vi "Compile Engine Data.vi"(8 "error in (no error)":errorcluster, 11 "Device Item Ref in":T1 format="%.0x") -> (0 "error out":errorcluster)   [LabVIEW 2023, in "NI 272x Resistive Simulation Custom Device Configuration.lvlib"]
uses:
  NI 272x Resistive Simulation Custom Device Configuration.lvlib
  <vilib>/NI VeriStand/Custom Device API/Custom Device Item Ref.ctl
  Controls/Compiled Engine Data.ctl
  Controls/Compiled HW Channel.ctl
  Controls/Channel Mode.ctl
  <instrlib>/ni272xReferenceVIs/ni272xReferenceVIs.llb/ni272x Callendar-Van Dusen RTD Parameters.ctl
  Controls/Compiled Connect Channel.ctl
  Globals/Names.vi
  <vilib>/NI VeriStand/Custom Device Tools/Custom Device Utility Library/NI VeriStand - Search for Item by Name.vi
  <vilib>/NI VeriStand/Custom Device API/Get Item Property (String).vi
  <vilib>/NI VeriStand/Custom Device API/Get Item Property (Double).vi
  <vilib>/NI VeriStand/Custom Device API/Set Item Property (Variant).vi
  <vilib>/NI VeriStand/Custom Device Tools/Custom Device Utility Library/Custom Device Utility Library.lvlib
  <vilib>/NI VeriStand/Custom Device API/Custom Device API.lvlib
  NI 272x Resistive Simulation Custom Device Shared.lvlib
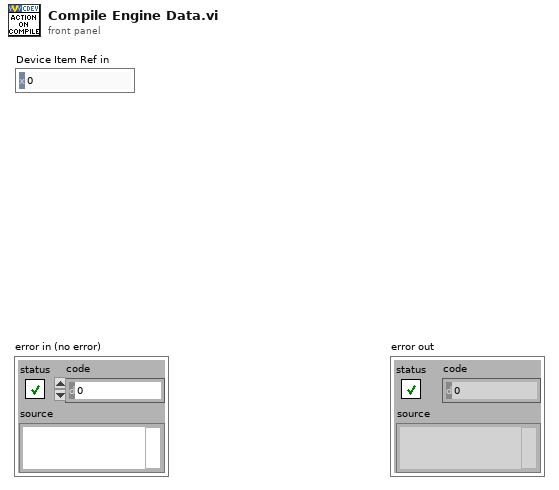
[diagram p1: front panel]
types:
  T1 = typedef "Custom Device API.lvlib/Custom Device Item Ref.ctl" = u64
  T2 = typedef "NI 272x Resistive Simulation Custom Device Shared.lvlib/Compiled Engine Data.ctl" = cluster{"HW Chns":T3[], "Con Chns":T6[], "Err Idx":i32, "Late Idx":i32, "Dur Idx":i32, "DevName":string, "CD In Size":i32, "CD Out Size":i32, "TL dt":i64}
  T3 = typedef "NI 272x Resistive Simulation Custom Device Shared.lvlib/Compiled HW Channel.ctl" = cluster{"Mode":T4, "RTD":T5, "Desired Idx":i32, "Actual Idx":i32, "Last Des Val":dbl, "HW CH":string}
  T4 = typedef "NI 272x Resistive Simulation Custom Device Shared.lvlib/Channel Mode.ctl" = enum16{"Resistance", "RTD Temperature"}
  T5 = typedef "ni272x Callendar-Van Dusen RTD Parameters.ctl" = cluster{"A":dbl, "B":dbl, "C":dbl, "R0":dbl}
  T6 = typedef "NI 272x Resistive Simulation Custom Device Shared.lvlib/Compiled Connect Channel.ctl" = cluster{"Chn Idx":i32, "HW CH":string, "Is Con":bool, "HW CH+1":string}
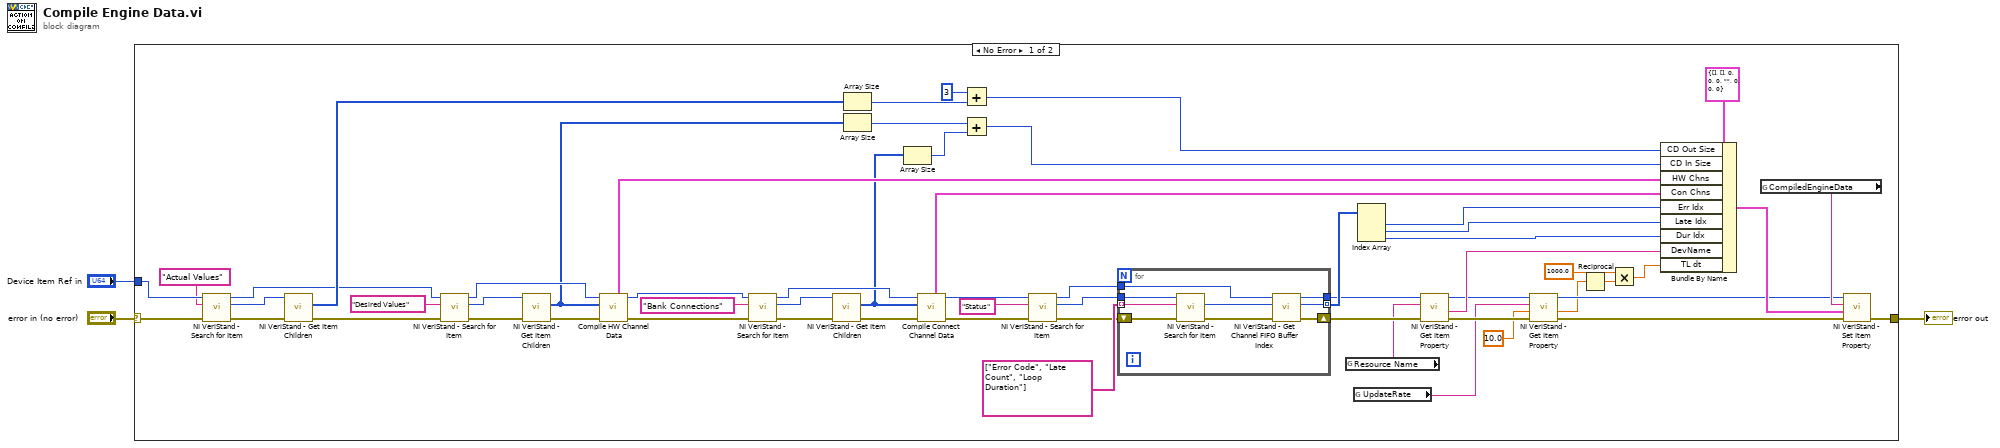
[diagram p0: block diagram]
diagram:
  n1 = case shown="No Error" "error in (no error)" {
    selector: "error in (no error)" -> [w62 w72]
    tunnel: [w34 w72] -> w2
    tunnel: "Device Item Ref in" -> [w10 _]
    frame No Error {
      n2 = call-poly <vilib>:"NI VeriStand - Search for Item.vi"("error in"=w62, "Item Name"="Actual Values", "Section Ref in"=w10) -> ("error out"=w11:errorcluster, "Item Ref"=w5:T1, "Section Ref out"=w4:T1)  [unwired: 5 in, 1 out]
      n3 = call <vilib>:"NI VeriStand - Get Item Children.vi"("error in (no error)"=w11, "Item Ref in"=w5) -> ("error out"=w8:errorcluster, "Child Refs"=w7:T1[])  [unwired: 6 in, 2 out]
      n4 = call-poly <vilib>:"NI VeriStand - Search for Item.vi"("error in"=w8, "Item Name"="Desired Values", "Section Ref in"=w4) -> ("error out"=w60:errorcluster, "Item Ref"=w59:T1, "Section Ref out"=w57:T1)  [unwired: 5 in, 1 out]
      n5 = call <vilib>:"NI VeriStand - Get Item Children.vi"("error in (no error)"=w60, "Item Ref in"=w59) -> ("error out"=w58:errorcluster, "Child Refs"=w27:T1[])  [unwired: 6 in, 2 out]
      n6 = call "Compile HW Channel Data.vi"("error in (no error)"=w58, "Desired Values Refs"=w27, "Device ref"=w57) -> ("error out"=w53:errorcluster, "Device ref dup"=w52:T1, "Compiled HW Channels"=w55:T3[])  [unwired: 6 in]
      n7 = call-poly <vilib>:"NI VeriStand - Search for Item.vi"("error in"=w53, "Item Name"="Bank Connections", "Section Ref in"=w52) -> ("error out"=w51:errorcluster, "Item Ref"=w49:T1, "Section Ref out"=w48:T1)  [unwired: 5 in, 1 out]
      n8 = call <vilib>:"NI VeriStand - Get Item Children.vi"("error in (no error)"=w51, "Item Ref in"=w49) -> ("error out"=w50:errorcluster, "Child Refs"=w26:T1[])  [unwired: 6 in, 2 out]
      n9 = Array Size(array=w7) -> (size(s)=w6:i32)
      n10 = Array Size(array=w27) -> (size(s)=w25:i32)
      n11 = Array Size(array=w26) -> (size(s)=w24:i32)
      n12 = call "Compile Connect Channel Data.vi"("error in (no error)"=w50, "Connect Chan Refs"=w26, "Device ref"=w48) -> ("error out"=w46:errorcluster, "Device ref dup"=w45:T1, "Compiled HW Channels"=w47:T6[])  [unwired: 6 in]
      n13 = Add(x=3, y=w6) -> (x+y=w21:i32)
      n14 = Add(x=w25, y=w24) -> (x+y=w23:i32)
      n15 = call-poly <vilib>:"NI VeriStand - Search for Item.vi"("error in"=w46, "Item Name"="Status", "Section Ref in"=w45) -> ("error out"=w42:errorcluster, "Item Ref"=w41:T1, "Section Ref out"=w40:T1)  [unwired: 5 in, 1 out]
      n16 = for {
        tunnel: string[] ["Error Code", "Late Count", "Loop Duration"] -> [w71] mode=indexing
        tunnel: w41 -> [w69]
        shift-right: [w65] -> w35
        shift-left: w42 -> [w70]
        tunnel: w40 -> [w67]
        tunnel: [w64] -> w39 mode=indexing
        tunnel: [w63] -> w30
        n17 = call-poly <vilib>:"NI VeriStand - Search for Item.vi"("error in"=w70, "Item Name"=w71, "Section Ref in"=w69) -> ("error out"=w68:errorcluster, "Item Ref"=w66:T1)  [unwired: 5 in, 2 out]
        n18 = call <vilib>:"NI VeriStand - Get Channel FIFO Buffer Index.vi"("error in"=w68, "Channel Ref"=w66, "Device Ref in"=w67) -> ("error out"=w65:errorcluster, "Channel FIFO Buffer Index"=w64:i32, "Device Ref out"=w63:T1)  [unwired: 4 in, 2 out]
      }
      n19 = global read "Names.vi" "Resource Name"() -> (w29:string)
      n20 = global read "Names.vi" "UpdateRate"() -> (w17:string)
      n21 = Index Array(array=w39) -> (element #1=w38:i32, element #2=w37:i32, element #3=w36:i32)  [unwired: 3 in]
      n22 = call-poly <vilib>:"NI VeriStand - Get Item Property.vi"("error in (no error)"=w35, "Property Name"=w29, "Item Ref in"=w30) -> ("error out"=w31:errorcluster, "Value"=w28:string, "Item Ref out"=w19:T1)  [unwired: 5 in, 1 out]
      n23 = call-poly <vilib>:"NI VeriStand - Get Item Property.vi"("error in (no error)"=w31, "Default Value"=10.0, "Property Name"=w17, "Item Ref in"=w19) -> ("error out"=w20:errorcluster, "Value"=w13:dbl, "Item Ref out"=w18:T1)  [unwired: 4 in, 1 out]
      n24 = Reciprocal(x=w13) -> (1/x=w15:dbl)
      n25 = Multiply(x=1000.0, y=w15) -> (x*y=w12:dbl)
      n26 = Bundle By Name(cluster=T2 {"HW Chns"=[], "Con Chns"=[], "Err Idx"=0, "Late Idx"=0, "Dur Idx"=0, "DevName"="", "CD In Size"=0, "CD Out Size"=0, "TL dt"=0} ("Engine Run Time Data"), "CD Out Size"=w21, "CD In Size"=w23, "HW Chns"=w55, "Con Chns"=w47, "Err Idx"=w38, "Late Idx"=w37, "Dur Idx"=w36, "DevName"=w28, "TL dt"=w12) -> (w32:T2)
      n27 = global read "Names.vi" "CompiledEngineData"() -> (w33:string)
      n28 = call-poly <vilib>:"NI VeriStand - Set Item Property.vi"("error in (no error)"=w20, "Value"=w32, "Property Name"=w33, "Item Ref in"=w18) -> ("error out"=w34:errorcluster)  [unwired: 5 in, 2 out]
    }
    frame Error {
    }
  }
  "error out" <- w2
